vi "n timed jump abs.vi"(7 "time":dbl, 8 "error in (no error)":errorcluster, 9 "y":i16, 10 "x":i16, 11 "n":u16) -> (0 "error out":errorcluster)   [LabVIEW 2015, in "SCANalone4x64.lvlib"]
doc: "__declspec(dllimport) void __stdcall n_timed_jump_abs(unsigned short n, short x, short y, double time);"
uses:
  <userlib>/SCANalone4x64/SCANalone4x64.lvlib
  <userlib>/SCANalone4x64/SCANalone4x64.dll
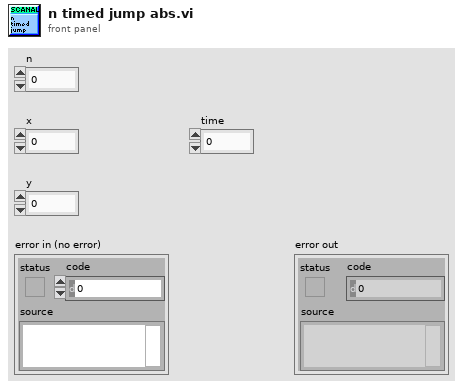
[diagram p1: front panel]
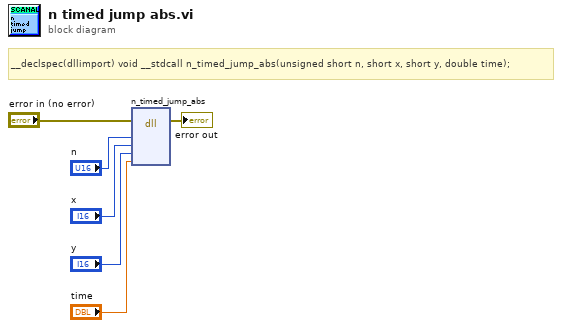
[diagram p0: block diagram]
diagram:
  # "__declspec(dllimport) void __stdcall n_timed_jump_abs(unsigned short n, short x, short y, double time);"
  n1 = dll-call lib="C:/Program Files/National Instruments/LabVIEW 2015/user.lib/SCANalone4x64/SCANalone4x64.*" fn="n_timed_jump_abs"(error in="error in (no error)", "n"="n", "x"="x", "y"="y", "time"="time") -> (error out=→"error out":errorcluster)  [unwired: 7 in, 1 out]
